vi "MALT132 IOPS.vi"() -> ()   [LabVIEW 2018]
uses:
  <instrlib>/AltonTech MALT/AltonTech MALT200817.lvlib
panel:
  in  "Average":u32
  out "IOPS":u32
  out "Total Time":u32
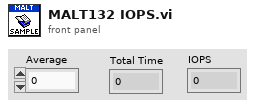
[diagram p1: front panel]
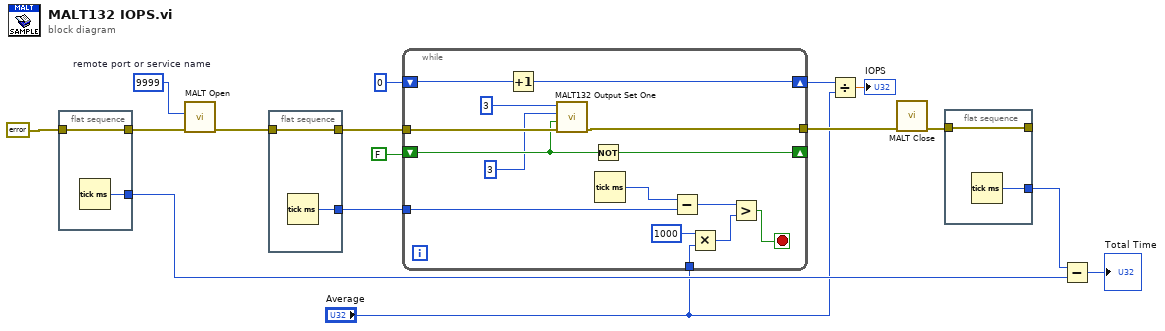
[diagram p0: block diagram]
diagram:
  w14 = u16 9999  # remote port or service name
  n1 = flat-sequence {
    tunnel: errorcluster {"status"=FALSE, "code"=0, "source"=""} ("error in (no error)") -> [w18]
    tunnel: [w18] -> w15
    tunnel: [w17] -> w13
    frame #0 {
      n2 = Tick Count (ms)() -> (millisecond timer value=w17:u32)
    }
  }
  n3 = call <instrlib>:"MALT Open.vi"("error in"=w15, 10:w14) -> ("error out"=w8:errorcluster)  [unwired: 9 in]
  n4 = flat-sequence {
    tunnel: w8 -> [w20]
    tunnel: [w20] -> w7
    tunnel: [w19] -> w6
    frame #0 {
      n5 = Tick Count (ms)() -> (millisecond timer value=w19:u32)
    }
  }
  n6 = while {
    tunnel: [w29] -> w9
    tunnel: w7 -> [w28]
    tunnel: w6 -> [w34]
    shift-right: [w31] -> w3
    shift-left: u32 0 ("x") -> [w32]
    shift-right: [w26] -> _
    shift-left: FALSE ("State") -> [w27]
    tunnel: "Average" -> [w21]
    stop <- w33 stop-if-true
    n7 = Increment(x=w32) -> (x+1=w31:u32)
    n8 = call <instrlib>:"MALT132 Output Set One.vi"("error in"=w28, "State"=w27, "Relay Num"=3, "Address"=3) -> ("error out"=w29:errorcluster)  [unwired: 7 in]
    n9 = Not(x=w27) -> (.not. x?=w26:bool)
    n10 = Tick Count (ms)() -> (millisecond timer value=w35:u32)
    n11 = Subtract(x=w35, y=w34) -> (x-y=w30:u32)
    n12 = Multiply(x=u32 1000, y=w21) -> (x*y=w23:u32)
    n13 = Greater?(x=w30, y=w23) -> (0:w33:bool)
  }
  n14 = Divide(x=w3, y="Average") -> (x/y=→"IOPS":dbl)
  n15 = call <instrlib>:"MALT Close.vi"("error in"=w9) -> ("error out"=w11:errorcluster)  [unwired: 10 in]
  n16 = flat-sequence {
    tunnel: w11 -> [w37]
    tunnel: [w37] -> _
    tunnel: [w36] -> w10
    frame #0 {
      n17 = Tick Count (ms)() -> (millisecond timer value=w36:u32)
    }
  }
  n18 = Subtract(x=w10, y=w13) -> (x-y=→"Total Time":u32)
